vi "Set Enum Control Strings.vi"(8 "error in":errorcluster, 10 "Enum values":string, 11 "Enum Refnum in":refnum<vi>) -> (0 "error out":errorcluster, 3 "Enum Refnum out":refnum<vi>)   [LabVIEW 2019, in "gRPC Template Creation Utility.lvlib"]
uses:
  gRPC Template Creation Utility.lvlib
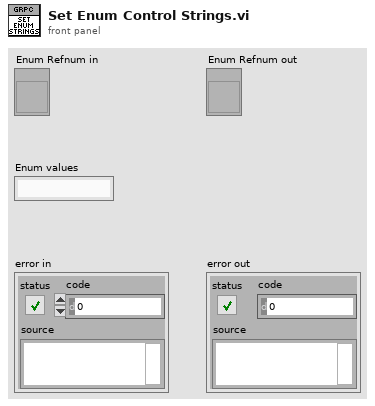
[diagram p1: front panel]
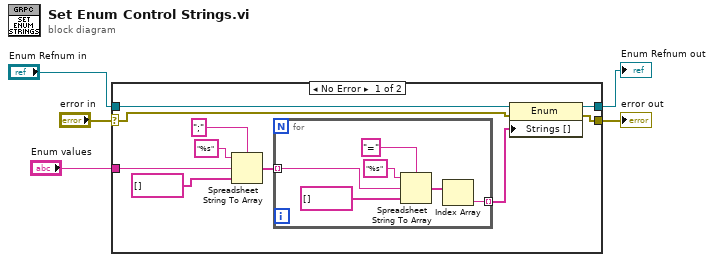
[diagram p0: block diagram]
diagram:
  n1 = case shown="No Error" "error in" {
    selector: "error in" -> [w11 w23]
    tunnel: "Enum Refnum in" -> [w15 w22]
    tunnel: "Enum values" -> [w14 _]
    tunnel: [w12 w23] -> w4
    tunnel: [w8 w22] -> w1
    frame No Error {
      n2 = Spreadsheet String To Array(delimiter (Tab)=";", format string="%s", spreadsheet string=w14, array type (2D Dbl)=string[] []) -> (array=w7:string[])
      n3 = for {
        tunnel: w7 -> [w17] mode=indexing
        tunnel: [w16] -> w6 mode=indexing
        n4 = Spreadsheet String To Array(delimiter (Tab)="=", format string="%s", spreadsheet string=w17, array type (2D Dbl)=string[] []) -> (array=w18:string[])
        n5 = Index Array(array=w18) -> (element=w16:string)  [unwired: 1 in]
      }
      n6 = property class="Enum"(reference=w15, error in=w11, "Strings []"=w6) -> (reference out=w8:refnum<vi>, error out=w12:errorcluster)
    }
    frame Error {
    }
  }
  "error out" <- w4
  "Enum Refnum out" <- w1
